vi "列表框test.vi"() -> ()   [LabVIEW 2019, in "test.lvlib"]
uses:
  test.lvlib
panel:
  out "数值":i32
  out "选中行":i32
  out "活动行:活动行数":i32
  in  "列表框":i32(listbox)=13
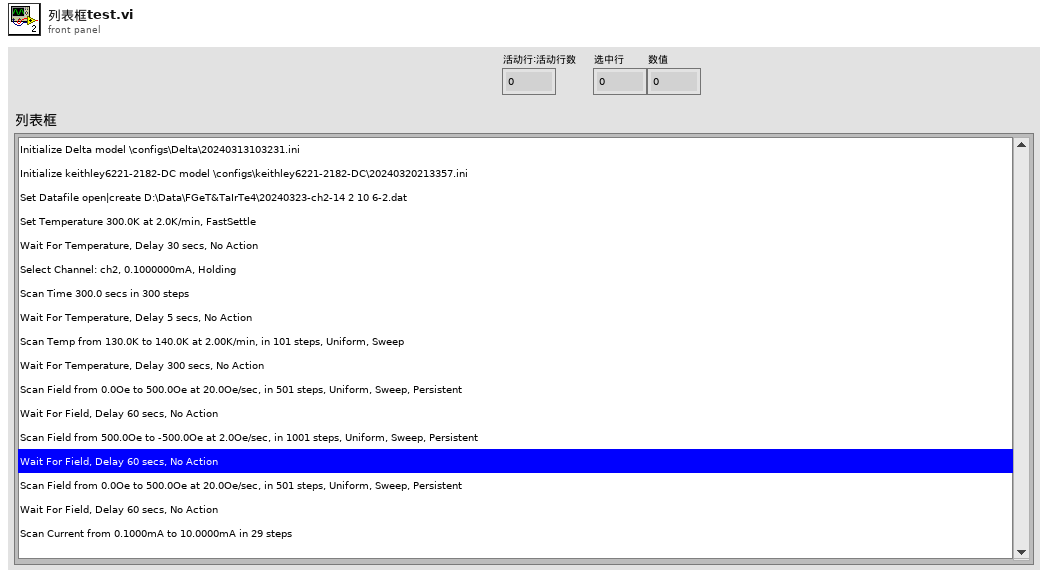
[diagram p1: front panel]
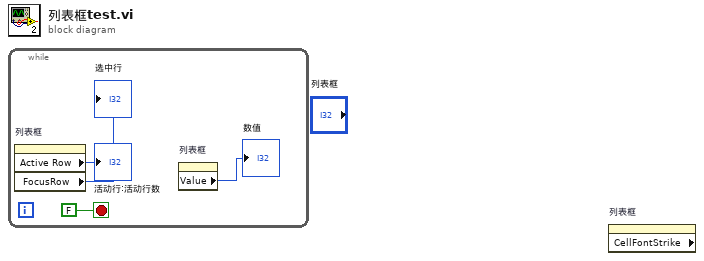
[diagram p0: block diagram]
diagram:
  n1 = while {
    stop <- FALSE stop-if-true
    n2 = property on="列表框" class="LstBox (严格)"() -> ("Active Row"=→"活动行:活动行数":i32, "FocusRow"=→"选中行":i32)  [unwired: 2 in, 2 out]
    n3 = property on="列表框" class="LstBox (严格)"() -> ("Value"=→"数值":i32)  [unwired: 2 in, 2 out]
  }
  n4 = property on="列表框" class="LstBox (严格)" props=["CellFontStrike"]() -> ()  [unwired: 2 in, 3 out]
